vi "niDTS GNSS GPS Rx RF Test UTIL Channel to Frequency.vi"(1 "Channel IN":T1) -> (0 "Frequency (Hz) OUT":dbl)   [LabVIEW 2014, in "niDTS GNSS.lvlib"]
uses:
  niDTS GNSS.lvlib
  Includes/niDTS GNSS GPS Rx RF Test INC Channel.ctl
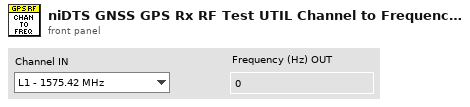
[diagram p1: front panel]
types:
  T1 = typedef "niDTS GNSS.lvlib/niDTS GNSS GPS Rx RF Test INC Channel.ctl" = enum16{"L1 - 1575.42 MHz", "L2 - 1227.60 MHz", "L5 - 1176.45 MHz"}
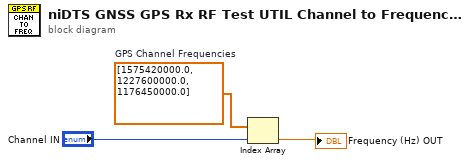
[diagram p0: block diagram]
diagram:
  w1 = dbl[] [1575420000.0, 1227600000.0, 1176450000.0]  # GPS Channel Frequencies
  n1 = Index Array(array=w1, index="Channel IN") -> (element=→"Frequency (Hz) OUT":dbl)
